vi "Prts Number.vi"(2 "Value from LPCA":string, 3 "Command":T1(ring)) -> (0 "Part Number":string, 1 "Index":i32)   [LabVIEW 2017]
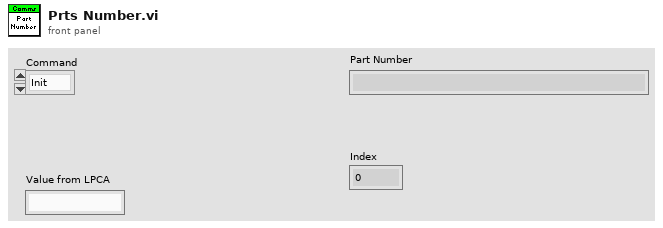
[diagram p1: front panel]
types:
  T1 = enum16{"Init", "Get Index", "Analyze", "Set VER", "Set TYPE"}
  T2 = cluster{"Hex Values":u8[], "Index":i32, "VER":string, "TYPE":string}
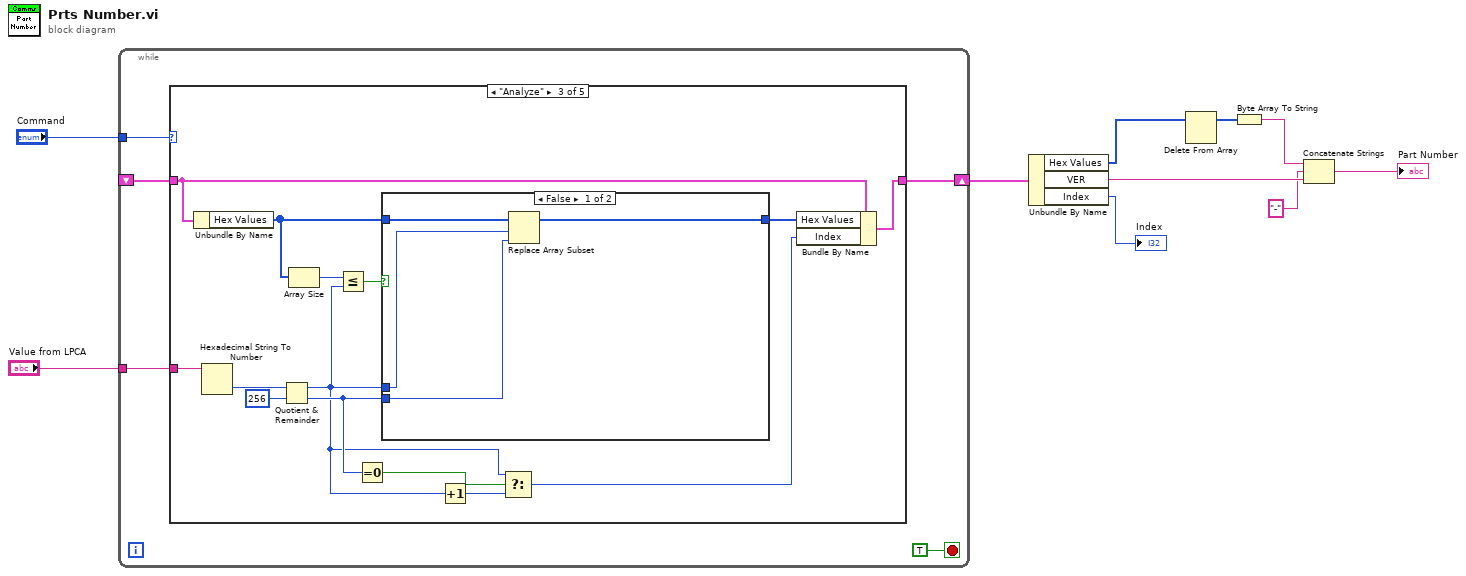
[diagram p0: block diagram]
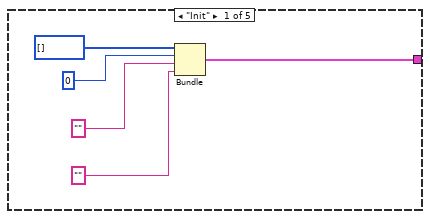
[diagram p2: hidden frame]
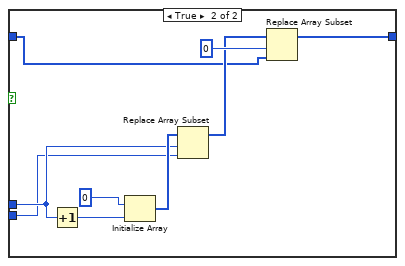
[diagram p4: hidden frame]
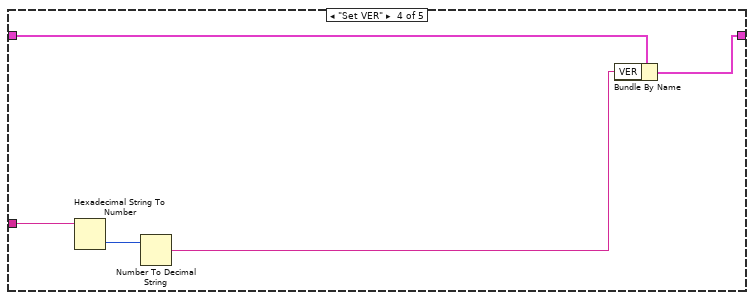
[diagram p5: hidden frame]
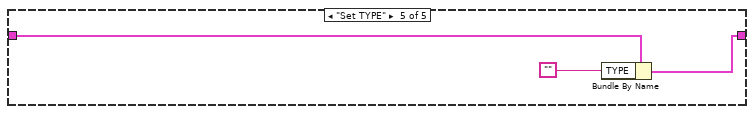
[diagram p6: hidden frame]
diagram:
  n1 = while {
    tunnel: "Command" -> [w15]
    tunnel: "Value from LPCA" -> [w14]
    shift-right: [w13] -> w8
    shift-left: _ -> [w12]
    stop <- TRUE stop-if-true
    n2 = case shown="\"Analyze\"" w15 {
      tunnel: w14 -> [_ _ w34 w53 _]
      tunnel: [w18 w21 w35 w50 w55] -> w13
      tunnel: w12 -> [_ w21 w31 w51 w56]
      frame "Init" {
        n3 = Bundle("Hex Values"=u8[] [], "Index"=0, "VER"="", "TYPE"="") -> (w18:T2)  [unwired: 1 in]
      }
      frame "Get Index" {
      }
      frame "Analyze" {
        n4 = Unbundle By Name(w31) -> ("Hex Values"=w28:u8[])
        n5 = Hexadecimal String To Number(string=w34) -> (number=w33:u32)  [unwired: 2 in, 1 out]
        n6 = Quotient & Remainder(x=w33, y=u32 256) -> (x-y*floor(x/y)=w22:u32, floor(x/y)=w26:u32)
        n7 = Array Size(array=w28) -> (size(s)=w30:i32)
        n8 = Less Or Equal?(x=w30, y=w22) -> (x <= y?=w29:bool)
        n9 = Equal To 0?(x=w26) -> (x = 0?=w23:bool)
        n10 = case shown="False" w29 {
          tunnel: w28 -> [w39 w40]
          tunnel: w22 -> [w37 w45]
          tunnel: w26 -> [w38 w44]
          tunnel: [w36 w42] -> w27
          frame False {
            n11 = Replace Array Subset(array=w39, new element=w38, index=w37) -> (w36:u8[])
          }
          frame True {
            n12 = Increment(x=w45) -> (x+1=w47:u32)
            n13 = Initialize Array(u8 0, w47) -> (w46:u8[])
            n14 = Replace Array Subset(array=w46, new element=w44, index=w45) -> (w41:u8[])
            n15 = Replace Array Subset(array=w41, new element=w40, index=0) -> (w42:u8[])
          }
        }
        n16 = Increment(x=w22) -> (x+1=w25:u32)
        n17 = Select(t=w22, s=w23, f=w25) -> (s? t:f=w24:u32)
        n18 = Bundle By Name(cluster=w31, "Hex Values"=w27, "Index"=w24) -> (w35:T2)
      }
      frame "Set VER" {
        n19 = Hexadecimal String To Number(string=w53) -> (number=w52:u32)  [unwired: 2 in, 1 out]
        n20 = Number To Decimal String(number=w52) -> (decimal integer string=w49:string)  [unwired: 1 in]
        n21 = Bundle By Name(cluster=w51, "VER"=w49) -> (w50:T2)
      }
      frame "Set TYPE" {
        n22 = Bundle By Name(cluster=w56, "TYPE"="") -> (w55:T2)
      }
    }
  }
  n23 = Unbundle By Name(w8) -> ("Hex Values"=w2:u8[], "VER"=w6:string, "Index"=→"Index":i32)
  n24 = Delete From Array(array=w2) -> (array with subset deleted=w1:u8[])  [unwired: 2 in, 1 out]
  n25 = Byte Array To String(unsigned byte array=w1) -> (string=w5:string)
  n26 = Concatenate Strings(w5, "-", w6) -> (→"Part Number":string)
